vi "error cluster.vi"() -> ()   [LabVIEW 2020]
uses:
  <vilib>/Utility/error.llb/Error Cluster From Error Code.vi
  <vilib>/ErrorRing/Error Ring.xnode
panel:
  out "error out":errorcluster
  out "error constant":errorcluster
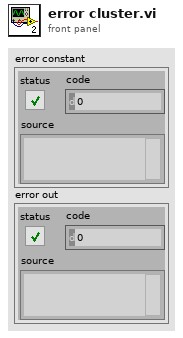
[diagram p1: front panel]
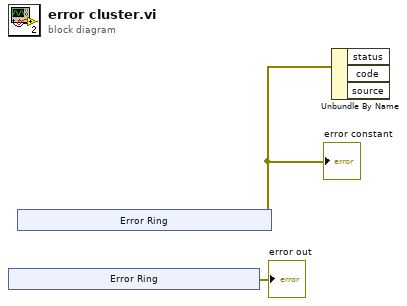
[diagram p0: block diagram]
diagram:
  n1 = xnode "Error Ring"() -> ("error out"=→"error out":errorcluster)
  n2 = xnode "Error Ring"() -> ("error out"=w2:errorcluster)
  "error constant" <- w2
  n3 = Unbundle By Name(w2) -> ()  [unwired: 3 out]
